vi "Main.vi"() -> ()   [LabVIEW 2016]
doc: "Main VI for the controls"
uses:
  Typedefs/StateDef_Enum.ctl
  <vilib>/Simulation/Scripting/Companion Diagram/SimConfigNode/SimParams.ctl
  <vilib>/Simulation/Scripting/Companion Diagram/SimConfigNode/_simSolvers.ctl
  <vilib>/Simulation/Implementation/Shared/SIMSCR Execution Mode.ctl
  <vilib>/Platform/TimedLoop/XDataNode/timing_clust.ctl
  <vilib>/Platform/TimedLoop/XDataNode/nitl_modes.ctl
  <vilib>/Platform/TimedLoop/XDataNode/wakeup.ctl
  <vilib>/Simulation/Param Hierarchy/Typedefs/SIMPH Param Control Actions.ctl
  <vilib>/Simulation/Implementation/Shared/SIM limit type.ctl
  <vilib>/Simulation/Scripting/Editor Utilities/SIM subVI tag data.ctl
  <vilib>/Simulation/Scripting/Editor Utilities/SIM subVI execution type.ctl
  <vilib>/Simulation/Implementation/Shared/NILVSim_ParamChanged.vi
  <vilib>/Simulation/Implementation/Shared/NILVSim_FinishedLate.vi
  <vilib>/Simulation/Implementation/Shared/NILVSIM_BeginStep.vi
  <vilib>/myRIO/Instrument Drivers/Onboard IO/AI/vis/Read.vi
  <vilib>/Simulation/Utility/Implementation/SIM SimulationParams.vi
  <vilib>/Simulation/ContinuousLinear/Implementation/NILVSim Transfer Function.llb/SIM Transfer Function Distributor (SISO).vi
  <vilib>/Simulation/Nonlinear/Implementation/NILVSim Saturation.llb/SIM Saturation (scalar).vi
  <vilib>/Simulation/ContinuousLinear/Implementation/NILVSim Integrator new.llb/SIM Integrator distributor (scalar).vi
  <vilib>/Simulation/Implementation/Shared/SIM Fire Discrete SubVI.vi
  <vilib>/Simulation/Utility/Implementation/SIM Halt.vi
  <vilib>/Simulation/ContinuousLinear/Implementation/NILVSim Transfer Function Direct.llb/SIM Transfer Function Direct (SISO).vi
  <vilib>/Simulation/SignalArithmetic/Implementation/NILVSim Gain.llb/SIM Gain (scalar).vi
  <vilib>/Simulation/ContinuousLinear/Implementation/NILVSim Integrator new.llb/SIM Integrator collector (scalar).vi
  <vilib>/Simulation/ContinuousLinear/Implementation/NILVSim Transfer Function.llb/SIM Transfer Function Collector (SISO).vi
  <vilib>/myRIO/Instrument Drivers/Onboard IO/AO/vis/Write.vi
  <vilib>/Simulation/Implementation/Shared/NILVSim_Manager.vi
  <vilib>/Utility/error.llb/Clear Errors.vi
  <vilib>/Simulation/Implementation/Shared/NILVSim_FinalizeModel.vi
  <vilib>/Simulation/Utility/Implementation/NILVSim SimulationParams (core).vi
  <vilib>/Simulation/Implementation/Shared/SIM Fire Discrete SubVI (Core).vi
  <vilib>/myRIO/Common/Instrument Driver Framework/myRIO v1.0/AI/vis/myRIO v1.0 Close AI.vi
  <vilib>/myRIO/Common/Instrument Driver Framework/myRIO v1.0/AO/vis/myRIO v1.0 Close AO.vi
  <vilib>/myRIO/Common/Instrument Driver Framework/myRIO v1.0/AI/vis/myRIO v1.0 Unreserve AI.vi
  <vilib>/myRIO/Common/Instrument Driver Framework/myRIO v1.0/AO/vis/myRIO v1.0 Unreserve AO.vi
  <vilib>/myRIO/Common/Instrument Driver Framework/myRIO v1.0/Resource Manager/vis/myRIO v1.0 Unreserve Channel List.vi
  <vilib>/myRIO/Common/Instrument Driver Framework/myRIO v1.0/AI/vis/myRIO v1.0 Build MUX Configuration AI.vi
  <vilib>/myRIO/Common/Instrument Driver Framework/myRIO v1.0/AO/vis/myRIO v1.0 Build MUX Configuration AO.vi
  <vilib>/myRIO/Common/Instrument Driver Framework/myRIO v1.0/Resource Manager/vis/myRIO v1.0 Unreserve Channel.vi
  <vilib>/myRIO/Common/Instrument Driver Framework/myRIO v1.0/Resource Manager/vis/myRIO v1.0 Build Mutex Name.vi
  <vilib>/Simulation/Implementation/Shared/SIM Unbundle Sim Info.vi
  <vilib>/Simulation/Implementation/Shared/SIMSH Read Queue.vi
  <vilib>/Simulation/Implementation/Shared/NILVSim_Initialize.vi
  <vilib>/Utility/error.llb/Error Cluster From Error Code.vi
  <vilib>/myRIO/Common/Instrument Driver Framework/myRIO v1.0/AI/vis/myRIO v1.0 Read AI.vi
  <vilib>/myRIO/Common/Instrument Driver Framework/myRIO v1.0/AO/vis/myRIO v1.0 Write AO.vi
  <vilib>/Simulation/Utility/Implementation/NILVSim Get Time and IsAcceptedStep.vi
  Components/Timing/Finished Late.vi
  <vilib>/Simulation/Implementation/Shared/NILVSim_GetModelError.vi
  <vilib>/Simulation/Implementation/Shared/SIM Bundle Sim Info.vi
  <vilib>/myRIO/Common/Instrument Driver Framework/Utilities/vis/Configuration Manager.vi
  <vilib>/myRIO/Common/Instrument Driver Framework/Utilities/vis/IO Manager.vi
  <vilib>/myRIO/Common/Instrument Driver Framework/myRIO v1.0/myRIO v1.0 Close.vi
  <vilib>/ErrorRing/Error Ring.xnode
  <vilib>/Simulation/Scripting/Companion Diagram/SimConfigNode/SimDog.xnode
  <vilib>/platform/TimedLoop/XDataNode/XDataNode.xnode
  <vilib>/Simulation/Implementation/XNodeFramework/SimXNode/SimX.xnode
  Components/Timing/Timing.lvlib
  <vilib>/myRIO/Instrument Drivers/Onboard IO/AI/AI.lvlib
  <vilib>/myRIO/Instrument Drivers/Onboard IO/AO/AO.lvlib
  <vilib>/Simulation/ContinuousLinear/Implementation/NILVSim Transfer Function.llb/SIM Transfer Function (SISO).vi
  <vilib>/Simulation/ContinuousLinear/Implementation/NILVSim Integrator new.llb/SIM Integrator (scalar).vi
  <vilib>/Platform/TimedLoop/XDataNode/XDNodeRunTimeDep.lvlib
  <vilib>/Simulation/Implementation/Shared/NI_SIM_Implementation.lvlib
panel:
  in  "Controller Params":enum32{"Page 1"}(tab)
  in  "Kp":dbl(slide)=1.0 scale=0.0..10.0 scale format="%#.1f"
  in  "Controller On?":bool
  out "Status":string
  in  "System Stop Button":bool
  in  "Ref. Gen.":enum32{"Analog In", "Manual", "Wave Gen"}(tab)=enum."Manual"
  in  "Ref. cmd.":dbl(slide) caption="Td (torque cmd.)" step=1.0 scale=-10.0..10.0 scale format="%#.1f"
  in  "Signal Cluster":T1={"phase"=0.0, "amplitude"=1.0, "frequency"=0.3, "offset"=1.0, "Signal"=enum."Sine"} {"offset" format="%0.2f"; "frequency" format="%0.2f"; "amplitude" format="%0.2f"; "phase" format="%0.2f"}
  in  "Loop Timing":enum32{"CD&Sim", "UI"}(tab)
  out "# Finished\nLate counter":dbl
  in  "CD&Sim\nLoop Rate (Hz)":dbl=4000.0 format="%#_4p"
  in  "UI Loop rate (Hz)":u32=20
  out "Waveform Chart":T2(graph)
  # "Please connect the Reference Signal \nto C/AI 0 of the myRIO"
  # "Control Loop Timing"
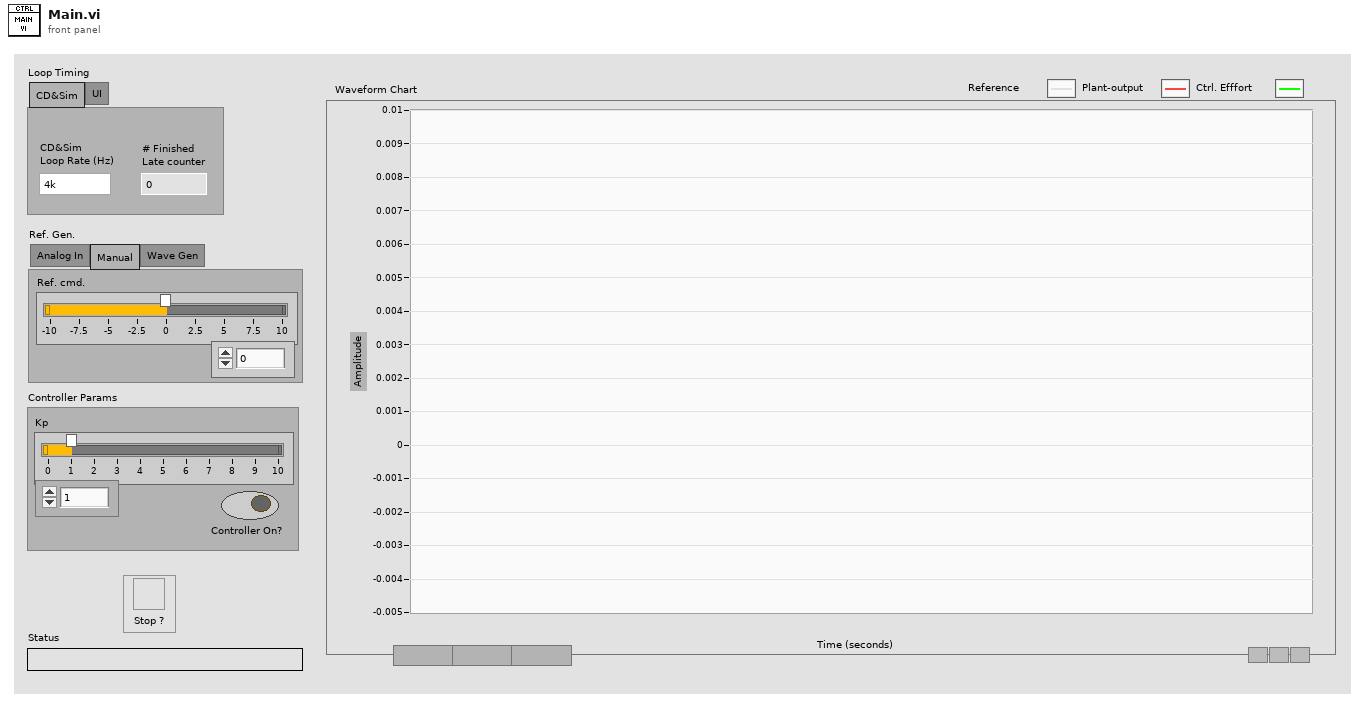
[diagram p1: front panel]
types:
  T1 = cluster{"phase":dbl, "amplitude":dbl, "frequency":dbl, "offset":dbl, "Signal":enum16{"Sine", "Square", "Sawtooth", "Random"}}
  T2 = cluster{"Numeric":dbl, "Numeric":dbl, "Numeric":dbl}
  T3 = typedef "StateDef_Enum.ctl" = enum16{"Initialize", "Wait", "Shutdown"}
  T4 = typedef "AI.lvlib/AI Reference.ctl" = cluster{"myRIO Reference":T5, "AI Channels List":T9, "AI Scaling Constants List":T11}
  T5 = typedef "myRIO Generic Hardware Reference.ctl" = cluster{"myRIO Model":T6, "myRIO Hardware Reference":T7}
  T6 = typedef "Hardware Version Enum.ctl" = enum16{"Unknown", "myRIO-1900", "myRIO-1950", "roboRIO", "NI ELVIS RIO CM"}
  T7 = typedef "myRIO v1.0 Reference.ctl" = cluster{"Generic FPGA Reference":T8, "Allow multiple opens":bool}
  T8 = typedef "Generic FPGA Reference.ctl" = refnum<k20>
  T9 = typedef "AI Channels List.ctl" = T10[]
  T10 = typedef "AI Channels Enum.ctl" = enum16{"Not Connected", "AudioIn/Left", "AudioIn/Right", "C/AI0", "C/AI1", "A/AI0", "A/AI1", "A/AI2", "A/AI3", "B/AI0", "B/AI1", "B/AI2", "B/AI3", "AI/AI0", "AI/AI1", "AI/AI2", "AI/AI3"}
  T11 = typedef "Analog Scaling Constants List.ctl" = T12[]
  T12 = typedef "Analog Scaling Constants.ctl" = cluster{"LSB Weight (Volts)":dbl, "Offset (Volts)":dbl, "Signed?":bool}
  T13 = typedef "AO.lvlib/AO Reference.ctl" = cluster{"myRIO Reference":T5, "AO Channel List":T14, "AO Scaling Constant List":T11}
  T14 = typedef "AO Channels List.ctl" = T15[]
  T15 = typedef "AO Channels Enum.ctl" = enum16{"Not Connected", "AudioOut/Left", "AudioOut/Right", "C/AO0", "C/AO1", "A/AO0", "A/AO1", "B/AO0", "B/AO1"}
  T16 = cluster{"Double":dbl, "Numeric":dbl, "Double":dbl}
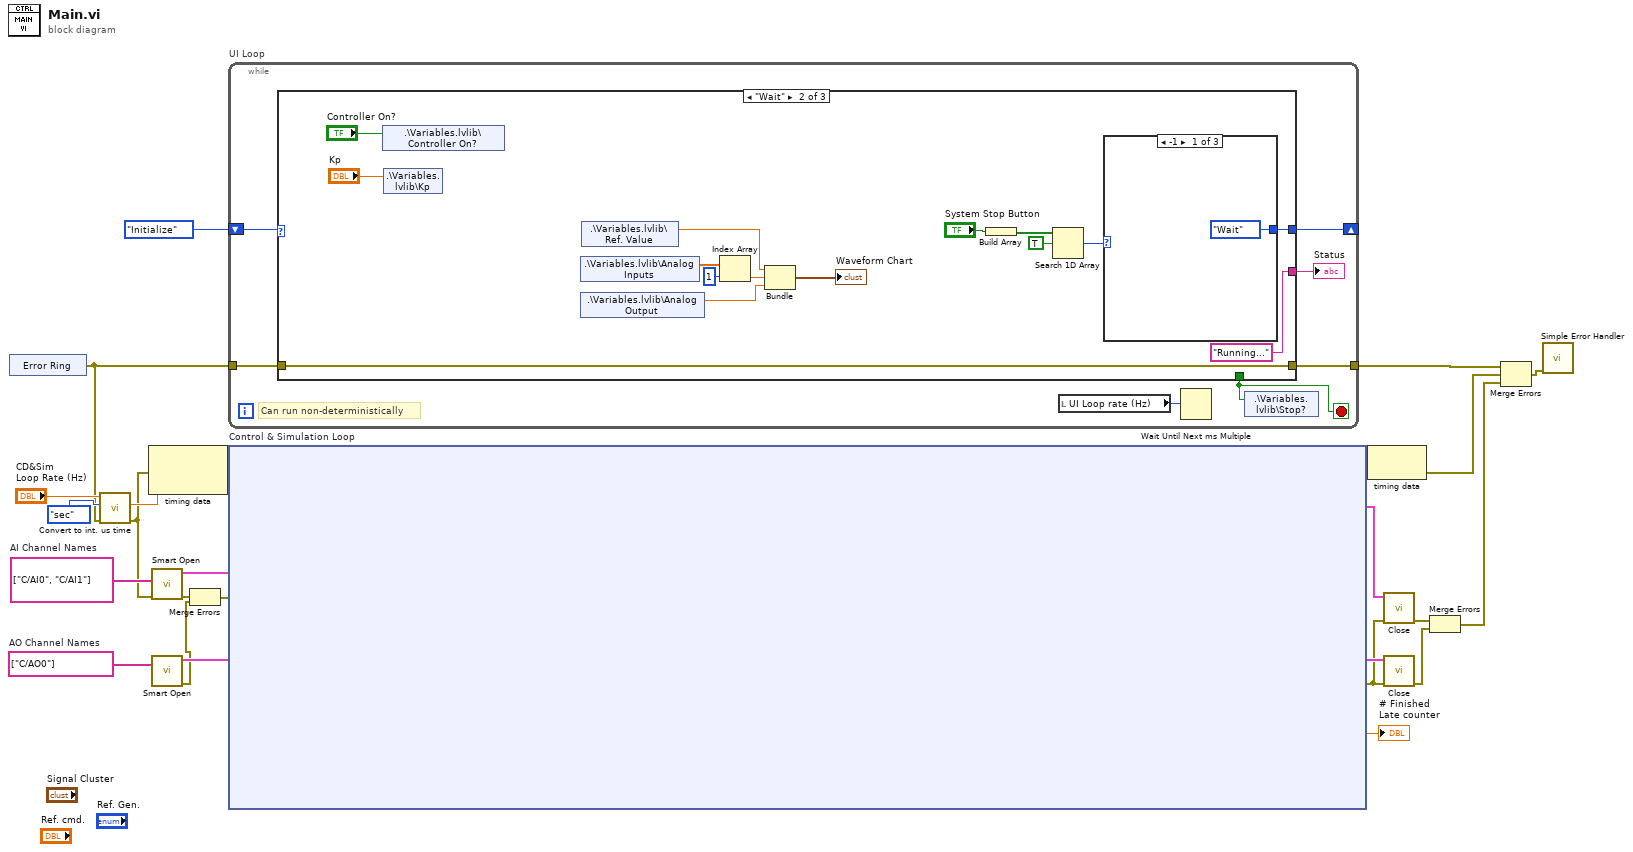
[diagram p0: block diagram]
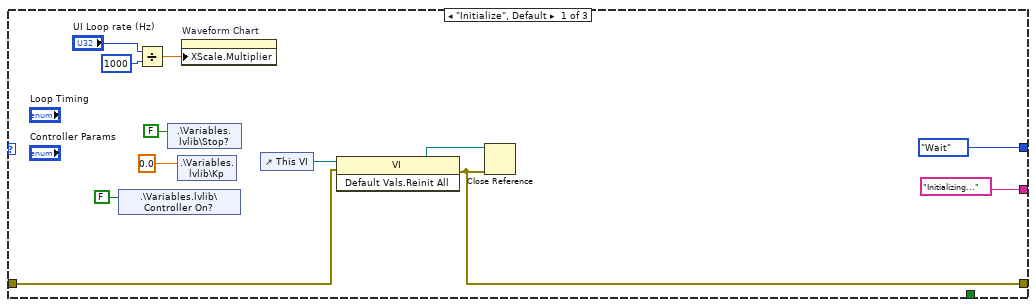
[diagram p2: hidden frame]
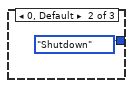
[diagram p3: hidden frame]
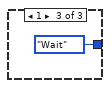
[diagram p4: hidden frame]
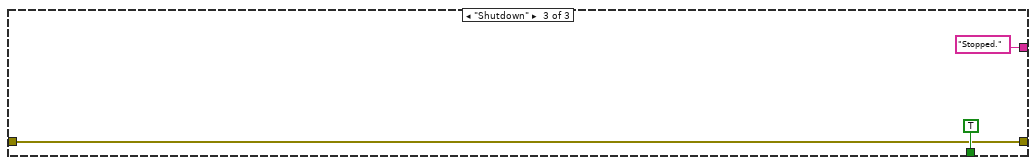
[diagram p5: hidden frame]
diagram:
  w11 = tag[] ["C/AO0"]  # AO Channel Names
  w12 = tag[] ["C/AI0", "C/AI1"]  # AI Channel Names
  n1 = xnode "Error Ring"() -> ("error out"=w18:errorcluster)
  n2 = call "Convert to int. us time.vi"("error in (no error)"=w18, "Int. Time Unit"=enum16{"sec", "us", "ms"}."sec", "Sample rate (Hz)"="CD&Sim\nLoop Rate (Hz)") -> ("error out"=w7:errorcluster, "Int.  time [unit]"=w20:dbl)  [unwired: 6 in, 1 out]
  n3 = node-c288(w7, w20) -> (w24:variant)
  n4 = call <vilib>:"Smart Open.vi"("error in (no error)"=w7, "Channel Names"=w12) -> ("error out"=w14:errorcluster, "AI Ref Out"=w15:T4)  [unwired: 8 in]
  n5 = call <vilib>:"Smart Open.vi"("Channel Names"=w11) -> ("error out"=w8:errorcluster, "AO Ref Out"=w10:T13)  [unwired: 9 in]
  n6 = Merge Errors(w14, w8) -> (w9:errorcluster)
  n7 = while "UI Loop" {
    shift-right: [w31] -> _
    shift-left: StateDef_Enum."Initialize" ("State defining Enum") -> [w32]
    tunnel: w18 -> [w28]
    tunnel: [w27] -> w17
    stop <- w30 stop-if-true
    # "Can run non-deterministically"
    n8 = case shown="\"Wait\"" w32 {
      tunnel: [StateDef_Enum."Wait" ("State defining Enum") w56 _] -> w31
      tunnel: [_ _ TRUE] -> w30
      tunnel: w28 -> [w37 w54 w64]
      tunnel: [w36 w54 w64] -> w27
      tunnel: ["Initializing..." ("Status") "Running..." ("Status") "Stopped." ("Status")] -> w26
      frame "Initialize", Default {
        n9 = shared-variable ".\\Variables.lvlib\\Controller On?"(FALSE ("Controller On?")) -> ()  [unwired: 1 in, 1 out]
        n10 = Divide(x="UI Loop rate (Hz)", y=u32 1000) -> (x/y=w41:dbl)
        n11 = shared-variable ".\\Variables.lvlib\\Stop?"(FALSE ("Stop?")) -> ()  [unwired: 1 in, 1 out]
        n12 = shared-variable ".\\Variables.lvlib\\Kp"(0.0 ("Kp")) -> ()  [unwired: 1 in, 1 out]
        n13 = property on="Waveform Chart" class="WFChart (strict)"("XScale.Multiplier"=w41) -> ()  [unwired: 2 in, 2 out]
        n14 = control-ref of="This VI"() -> (w39:refnum<vi>)
        n15 = invoke class="VI" method="Default Vals.Reinit All"(reference=w39, error in=w37) -> (reference out=w38:refnum<vi>, error out=w36:errorcluster)  [unwired: 1 in, 1 out]
        n16 = Close Reference(reference=w38, error in (no error)=w36) -> ()  [unwired: 1 out]
      }
      frame "Wait" {
        n17 = shared-variable ".\\Variables.lvlib\\Controller On?"("Controller On?") -> ()  [unwired: 1 in, 1 out]
        n18 = shared-variable ".\\Variables.lvlib\\Kp"("Kp") -> ()  [unwired: 1 in, 1 out]
        n19 = shared-variable ".\\Variables.lvlib\\Analog Inputs"() -> (w53:dbl[])  [unwired: 1 in, 1 out]
        n20 = shared-variable ".\\Variables.lvlib\\Analog Output"() -> (w46:dbl)  [unwired: 1 in, 1 out]
        n21 = shared-variable ".\\Variables.lvlib\\Ref. Value"() -> (w47:dbl)  [unwired: 1 in, 1 out]
        n22 = Index Array(array=w53, index=1) -> (element=w49:dbl)
        n23 = Bundle("Double"=w47, "Numeric"=w49, "Double"=w46) -> (→"Waveform Chart":T16)  [unwired: 1 in]
        n24 = Build Array("System Stop Button") -> (w58:bool[])
        n25 = Search 1D Array(1D array=w58, element=TRUE) -> (index of element=w55:i32)  [unwired: 1 in]
        n26 = case shown="-1" w55 {
          tunnel: [StateDef_Enum."Wait" ("State defining Enum") StateDef_Enum."Shutdown" ("State defining Enum") StateDef_Enum."Wait" ("State defining Enum")] -> w56
          frame -1 {
          }
          frame 0, Default {
          }
          frame 1 {
          }
        }
      }
      frame "Shutdown" {
      }
    }
    "Status" <- w26
    n27 = local read "UI Loop rate (Hz)"() -> (w29:u32)
    n28 = Wait Until Next ms Multiple(millisecond multiple=w29) -> ()  [unwired: 1 out]
    n29 = shared-variable ".\\Variables.lvlib\\Stop?"(w30) -> ()  [unwired: 1 in, 1 out]
  }
  n30 = node-c254 "Control & Simulation Loop"(w24, w15, w9, w10) -> (w23:variant, →"# Finished\nLate counter":dbl, w6:T13, w4:errorcluster, w5:T4)
  n31 = node-c288(w23) -> (w13:errorcluster)
  n32 = call <vilib>:"Close.vi"("error in (no error)"=w4, "AI Ref In"=w5) -> ("error out"=w3:errorcluster)  [unwired: 9 in]
  n33 = call <vilib>:"Close.vi"("error in (no error)"=w4, "AO Ref In"=w6) -> ("error out"=w2:errorcluster)  [unwired: 9 in]
  n34 = Merge Errors(w3, w2) -> (w1:errorcluster)
  n35 = Merge Errors(w17, w13, w1) -> (w16:errorcluster)
  n36 = call <vilib>:"Simple Error Handler.vi"("error in (no error)"=w16) -> ()  [unwired: 4 in, 5 out]
